vi "ScanSteuerung_LoopItAll.vi"(3 "needed constants":cluster{"AD-clock":dbl, "GalvoCycle":dbl}={"AD-clock"=4000000.0, "GalvoCycle"=1e-05}, 4 "ScanSteuerung":T1=[{"Time [s]"=0.0, "action"=enum."Abs", "channel"=enum."GalvoX", "value (/s)"=-8.3466666667e-05}, {"Time [s]"=0.0, "action"=enum."Abs", "channel"=enum."GalvoY", "value (/s)"=6.7466666667e-05}, {"Time [s]"=0.0, "action"=enum."Inc", "channel"=enum."GalvoX", "value (/s)"=0.0888}, {"Time [s]"=0.0, "action"=enum."Inc", "channel"=enum."GalvoY", "value (/s)"=0.0}, {"Time [s]"=0.00119, "action"=enum."LoopStart", "channel"=enum."Loop", "value (/s)"=4.0}, {"Time [s]"=0.00119, "action"=enum."Abs", "channel"=enum."Digital", "value (/s)"=7.0}, {"Time [s]"=0.002, "action"=enum."Inc", "channel"=enum."GalvoX", "value (/s)"=-3.3095271315e-17}, {"Time [s]"=0.002, "action"=enum."Inc", "channel"=enum."GalvoY", "value (/s)"=-0.0818}, {"Time [s]"=0.0022, "action"=enum."Inc", "channel"=enum."GalvoX", "value (/s)"=-0.0888}, {"Time [s]"=0.0022, "action"=enum."Inc", "channel"=enum."GalvoY", "value (/s)"=0.0}, {"Time [s]"=0.00319, "action"=enum."Abs", "channel"=enum."Digital", "value (/s)"=5.0}, {"Time [s]"=0.0033900000000000002, "action"=enum."Abs", "channel"=enum."Digital", "value (/s)"=7.0}, {"Time [s]"=0.0042, "action"=enum."Inc", "channel"=enum."GalvoX", "value (/s)"=3.3095271315e-17}, {"Time [s]"=0.0042, "action"=enum."Inc", "channel"=enum."GalvoY", "value (/s)"=-0.0818}, {"Time [s]"=0.0044, "action"=enum."Inc", "channel"=enum."GalvoX", "value (/s)"=0.0888}, {"Time [s]"=0.0044, "action"=enum."Inc", "channel"=enum."GalvoY", "value (/s)"=0.0}, {"Time [s]"=0.00539, "action"=enum."Abs", "channel"=enum."Digital", "value (/s)"=5.0}, {"Time [s]"=0.00559, "action"=enum."LoopEnd", "channel"=enum."Loop", "value (/s)"=0.0}, {"Time [s]"=0.01879, "action"=enum."Abs", "channel"=enum."Digital", "value (/s)"=7.0}, {"Time [s]"=0.0196, "action"=enum."Inc", "channel"=enum."GalvoX", "value (/s)"=-3.3095271315e-17}, {"Time [s]"=0.0196, "action"=enum."Inc", "channel"=enum."GalvoY", "value (/s)"=-0.0818}, {"Time [s]"=0.0198, "action"=enum."Inc", "channel"=enum."GalvoX", "value (/s)"=-0.0888}, {"Time [s]"=0.0198, "action"=enum."Inc", "channel"=enum."GalvoY", "value (/s)"=0.0}, {"Time [s]"=0.02079, "action"=enum."Abs", "channel"=enum."Digital", "value (/s)"=5.0}, {"Time [s]"=0.02099, "action"=enum."Abs", "channel"=enum."Digital", "value (/s)"=7.0}, {"Time [s]"=0.0218, "action"=enum."Inc", "channel"=enum."GalvoX", "value (/s)"=0.0}, {"Time [s]"=0.0218, "action"=enum."Inc", "channel"=enum."GalvoY", "value (/s)"=0.0}, {"Time [s]"=0.02299, "action"=enum."Abs", "channel"=enum."Digital", "value (/s)"=0.0}], 5 "Times":u32=10) -> (0 "ScanSteuerungOut":T1=[{"Time [s]"=0.0, "action"=enum."Abs", "channel"=enum."SMoveTime", "value (/s)"=0.0008}, {"Time [s]"=0.0, "action"=enum."Abs", "channel"=enum."GalvoX", "value (/s)"=-0.0005000005}, {"Time [s]"=0.0, "action"=enum."Abs", "channel"=enum."GalvoY", "value (/s)"=-0.0005000005}, {"Time [s]"=0.0, "action"=enum."Abs", "channel"=enum."Galvo3", "value (/s)"=0.0}, {"Time [s]"=0.0, "action"=enum."LoopStart", "channel"=enum."Loop", "value (/s)"=10.0}, {"Time [s]"=0.0, "action"=enum."Inc", "channel"=enum."GalvoX", "value (/s)"=1.000001e-06}, {"Time [s]"=0.0, "action"=enum."Inc", "channel"=enum."GalvoY", "value (/s)"=0.0}, {"Time [s]"=0.0, "action"=enum."Inc", "channel"=enum."Galvo3", "value (/s)"=0.512}, {"Time [s]"=999.9999999999999, "action"=enum."Abs", "channel"=enum."Digital", "value (/s)"=1.0}, {"Time [s]"=999.9999999999999, "action"=enum."Inc", "channel"=enum."GalvoX", "value (/s)"=0.0}, {"Time [s]"=999.9999999999999, "action"=enum."Inc", "channel"=enum."GalvoY", "value (/s)"=6.25000625e-06}, {"Time [s]"=999.9999999999999, "action"=enum."Inc", "channel"=enum."Galvo3", "value (/s)"=0.0}, {"Time [s]"=1008.0, "action"=enum."Abs", "channel"=enum."Digital", "value (/s)"=0.0}, {"Time [s]"=1008.0, "action"=enum."Inc", "channel"=enum."GalvoX", "value (/s)"=-1.000001e-06}, {"Time [s]"=1008.0, "action"=enum."Inc", "channel"=enum."GalvoY", "value (/s)"=-0.0}, {"Time [s]"=1008.0, "action"=enum."Inc", "channel"=enum."Galvo3", "value (/s)"=-0.512}, {"Time [s]"=2008.0, "action"=enum."Abs", "channel"=enum."Digital", "value (/s)"=1.0}, {"Time [s]"=2008.0, "action"=enum."Inc", "channel"=enum."GalvoX", "value (/s)"=0.0}, {"Time [s]"=2008.0, "action"=enum."Inc", "channel"=enum."GalvoY", "value (/s)"=6.25000625e-06}, {"Time [s]"=2008.0, "action"=enum."Inc", "channel"=enum."Galvo3", "value (/s)"=0.0}, {"Time [s]"=2016.0, "action"=enum."Abs", "channel"=enum."Digital", "value (/s)"=0.0}, {"Time [s]"=2016.0, "action"=enum."LoopEnd", "channel"=enum."Loop", "value (/s)"=0.0}, {"Time [s]"=20160.0, "action"=enum."Inc", "channel"=enum."GalvoX", "value (/s)"=0.0}, {"Time [s]"=20160.0, "action"=enum."Inc", "channel"=enum."GalvoY", "value (/s)"=0.0}, {"Time [s]"=20160.0, "action"=enum."Inc", "channel"=enum."Galvo3", "value (/s)"=0.0}], 1 "Looptime (1 image)":dbl)   [LabVIEW 2011]
uses:
  ScanControl.ctl
  ScanControl_Action.ctl
  ScanControl_Channel.ctl
panel:
  out "next GalvoSyncTime T1+T2":dbl
  out "time of last galvo (t1)":dbl
  out "index last galvocomand":i32
  out "Total Time":dbl
  # "sync to galvotime and ADTime"
  # "vor inner loopstat biite ein digital=0!r"
  # "seems to work!!"
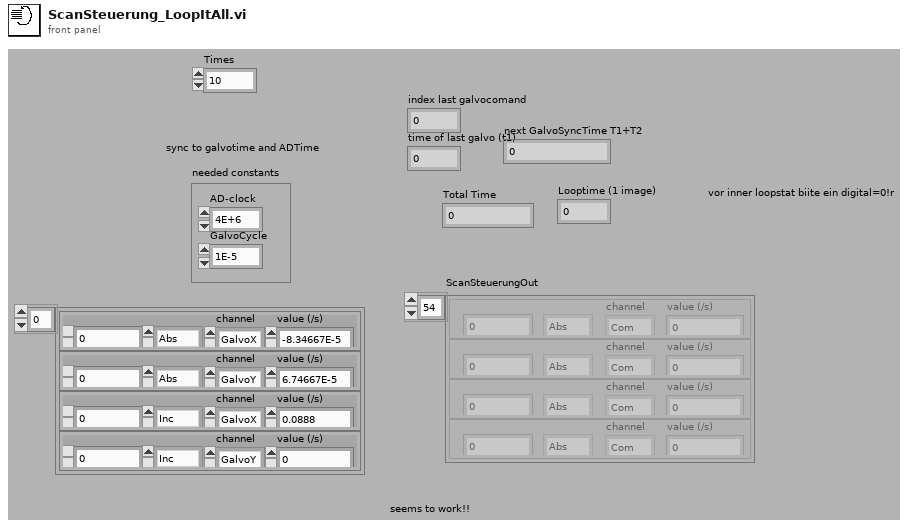
[diagram p1: front panel]
types:
  T1 = typedef "ScanControl.ctl" = cluster{"Time [s]":dbl, "action":T2, "channel":T3, "value (/s)":dbl}[]
  T2 = typedef "ScanControl_Action.ctl" = enum16{"Abs", "Rel", "Inc", "IncInc", "LoopStart", "LoopEnd", "WaitTriggerRising"}
  T3 = typedef "ScanControl_Channel.ctl" = enum16{"Com", "AnalogConfig", "AnalogValue", "GalvoX", "GalvoY", "Galvo3", "Galvo4", "Digital", "Free", "Loop", "SMoveTime", "Image1X", "Image1Y", "Image2X", "Image2Y"}
  T4 = enum16{"Com", "Digital", "Analog", "GalvoX", "GalvoY", "GalvoCCD", "Free1", "Free2", "Free3", "Loop", "SMoveTime", "Image1X", "Image1Y", "Image2X", "Image2Y"}
  T5 = enum16{"Com", "AnalogConfig", "AnalogValue", "GalvoX", "GalvoY", "Galvo3", "Galvo4", "Digital", "Free", "Loop", "SMoveTime", "Image1X", "Image1Y", "Image2X", "Image2Y"}
  T6 = enum16{"Abs", "Rel", "Inc", "IncInc", "LoopStart", "LoopEnd"}
  T7 = cluster{"Zeitpunkt [s]":dbl, "Wirkung":enum16{"Abs", "Rel", "Inc", "IncInc", "LoopStart", "LoopEnd"}, "Kanal":enum16{"Com", "AnalogConfig", "AnalogValue", "GalvoX", "GalvoY", "Galvo3", "Galvo4", "Digital", "Free", "Loop", "SMoveTime", "Image1X", "Image1Y", "Image2X", "Image2Y"}, "Wert (/s)":dbl}[]
  T8 = cluster{"Time [s]":dbl, "action":T2, "channel":T3, "value (/s)":dbl}
  T9 = cluster{"Time [s]":dbl, "Wirkung":enum16{"Abs", "Rel", "Inc", "IncInc", "LoopStart", "LoopEnd"}, "Kanal":enum16{"Com", "AnalogConfig", "AnalogValue", "GalvoX", "GalvoY", "Galvo3", "Galvo4", "Digital", "Free", "Loop", "SMoveTime", "Image1X", "Image1Y", "Image2X", "Image2Y"}, u32}
  T10 = cluster{dbl, "Wirkung":T2, "Kanal":enum16{"Com", "Digital", "Analog", "GalvoX", "GalvoY", "GalvoCCD", "Free1", "Free2", "Free3", "Loop", "SMoveTime", "Image1X", "Image1Y", "Image2X", "Image2Y"}, "Wert (/s)":dbl}
  T11 = cluster{"Time [s]":dbl, "action":T2, "Kanal":u16, "value (/s)":dbl}[]
  T12 = cluster{"Time [s]":dbl, "action":T2, "Kanal":u16, "value (/s)":dbl}
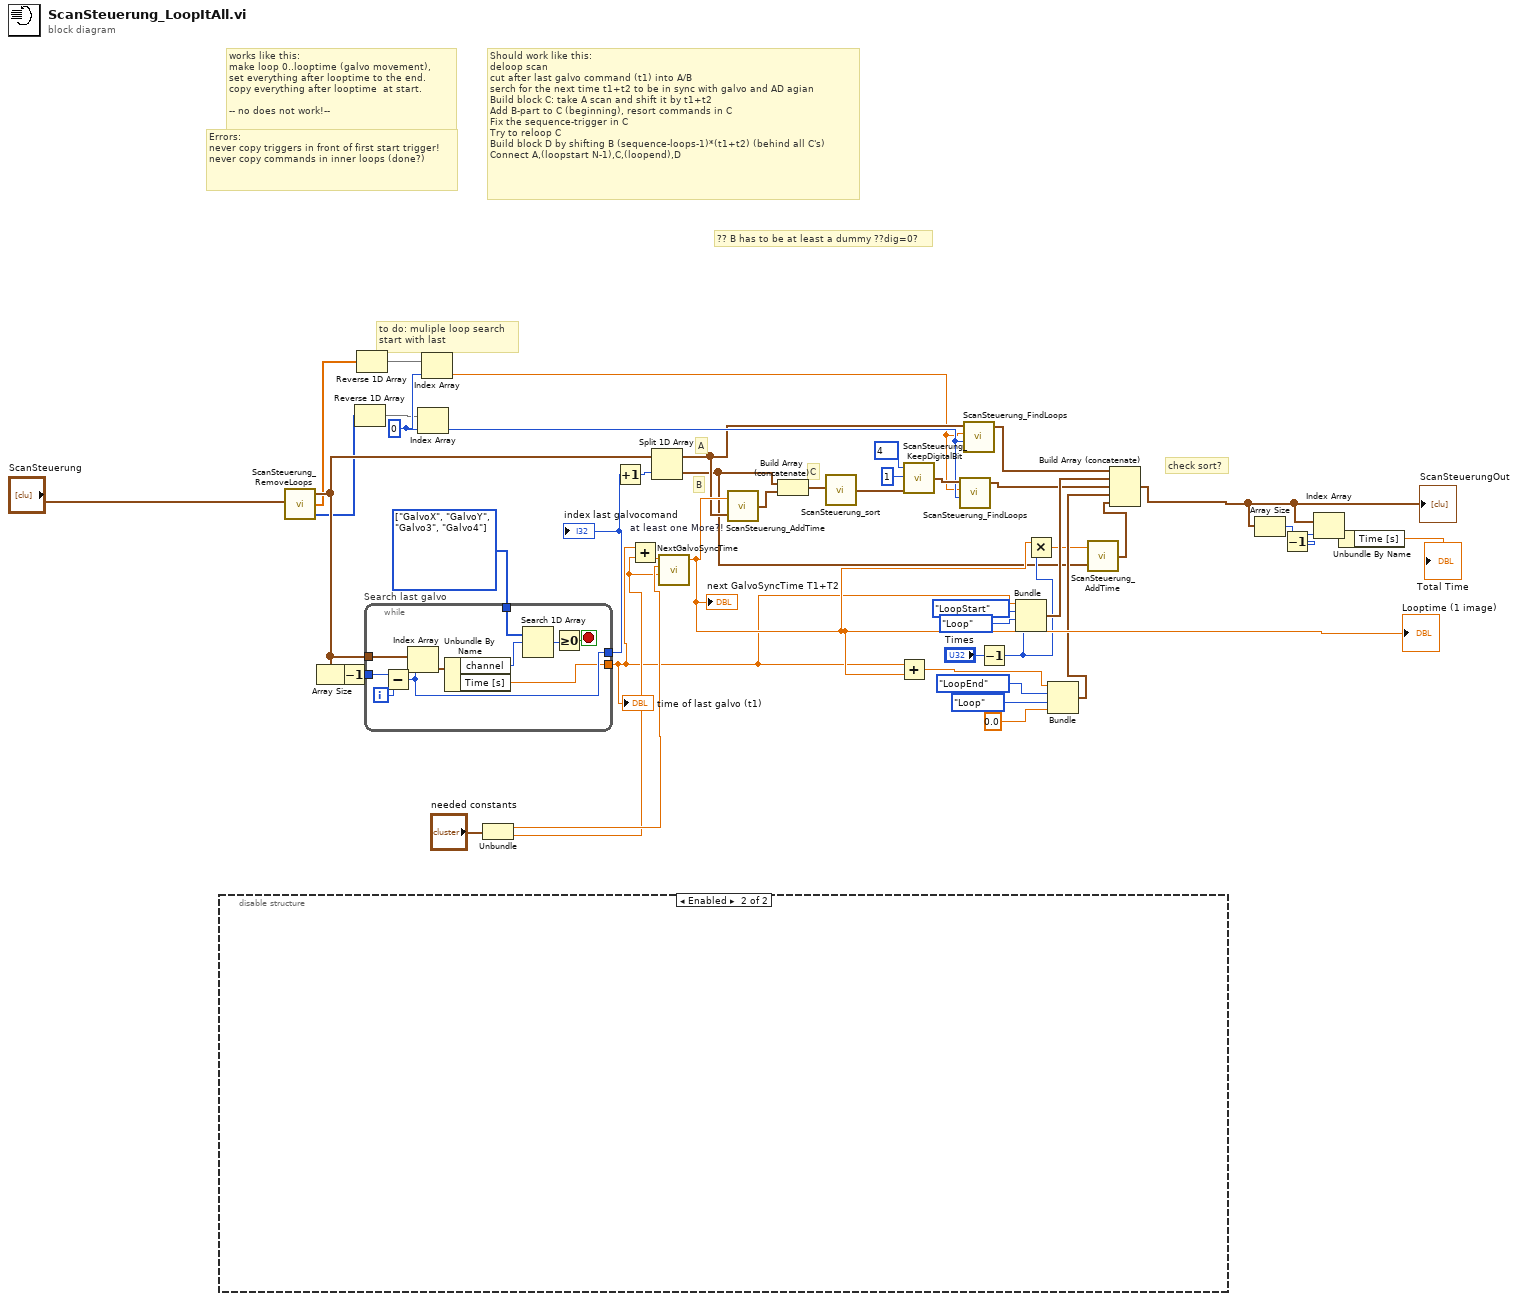
[diagram p0: block diagram]
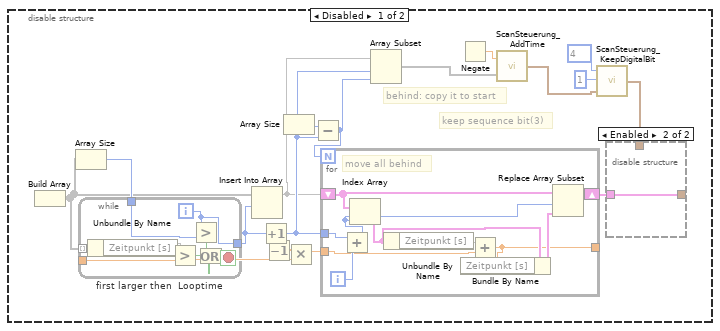
[diagram p2: hidden frame]
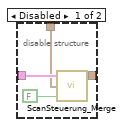
[diagram p3: hidden frame]
diagram:
  w3 = 0 ("index")
  w35 = T3[] [enum."GalvoX", enum."GalvoY", enum."Galvo3", enum."Galvo4"] items=["Com", "AnalogConfig", "AnalogValue", "GalvoX", "GalvoY", "Galvo3", "Galvo4", "Digital", "Free", "Loop", "SMoveTime", "Image1X", "Image1Y", "Image2X", "Image2Y"] ("1D array")
  # "check sort?"
  # "C"
  # "B"
  # "A"
  # "to do: muliple loop search\nstart with last"
  # "?? B has to be at least a dummy ??dig=0?"
  # "Errors:\nnever copy triggers in front of first start trigger!\nnever copy commands in inner loops (done?)"
  # "Should work like this:\ndeloop scan\ncut after last galvo command (t1) into A/B\nserch for the next time t1+t2 to be in sync with galvo and AD agian\nBuild block C: take A scan and shift it by t1+t2\nAdd B-part to C (beginning), resort commands in C\nFix the sequence-trigger in C\nTry to reloop C\nBuild block D by shifting B (sequence-loops-1)*(t1+t2) (behind all C's)\nConnect A,(loopstart N-1),C,(loopend),D"
  # "works like this: \nmake loop 0..looptime (galvo movement), \nset everything after looptime to the end.\ncopy everything after looptime  at start.\n\n-- no does not work!--"
  n1 = disable-structure shown="Enabled" {
    frame Disabled {
      # "keep sequence bit(3)"
      # "behind: copy it to start"
      n2 = Build Array() -> (w57:void[], w50:dbl, w51:dbl)
      n3 = Array Size(array=w57) -> (size(s)=w58:i32)
      n4 = Decrement() -> (x=w49:dbl, x-1=w56:dbl)
      n5 = Multiply(x=w56) -> (y=w64:dbl, x*y=w63:dbl)
      n6 = while "first larger then  Looptime" {
        tunnel: w57 -> [w93] mode=indexing
        tunnel: w64 -> [w91]
        tunnel: [w90] -> w54
        tunnel: w58 -> [w89]
        i -> [w90]
        stop <- w88 stop-if-true
        n7 = Unbundle By Name(w93) -> ("Zeitpunkt [s]"=w92)
        n8 = Greater?(x=w92, y=w91) -> (0:w87:bool)
        n9 = Greater?(x=w90, y=w89) -> (0:w86:bool)
        n10 = Or(x=w86, y=w87) -> (x .or. y?=w88:bool)
      }
      n11 = Insert Into Array(array=w57, index=w54) -> (w59, new element=w52:dbl)
      n12 = Increment(x=w54) -> (x+1=w61:i32)
      n13 = Array Size(array=w59) -> (size(s)=w53:i32)
      n14 = Subtract(x=w53, y=w61) -> (x-y=w60:i32)
      n15 = for {
        N: w60 -> [_]
        shift-right: [w82] -> w66
        shift-left: w59 -> [w83]
        tunnel: w63 -> [w80]
        tunnel: w61 -> [w85]
        tunnel: [w76] -> w55
        i -> [w84]
        # "move all behind"
        n16 = Add(x=w85, y=w84) -> (x+y=w77:i32)
        n17 = Index Array(array=w83, index=w77) -> (element=w79:cluster{})
        n18 = Unbundle By Name(w79) -> ("Zeitpunkt [s]"=w81)
        n19 = Add(x=w81, y=w80) -> (x+y=w76:dbl)
        n20 = Bundle By Name(cluster=w79, "Zeitpunkt [s]"=w76) -> (w78:cluster{})
        n21 = Replace Array Subset(array=w83, new element=w78, index=w77) -> (w82:cluster{}[])
      }
      n22 = Array Subset(array=w59, index=w61, length=w60) -> (w62:void[])
      n23 = Negate() -> (x=w48:dbl, -x=w65:dbl)
      n24 = call "ScanSteuerung_AddTime.vi"("ScanSteuerung"=w62, "Add Time"=w65) -> ("ScanSteuerungOut"=w67:T1)
      n25 = call "ScanSteuerung_KeepDigitalBit.vi"("ScanSteuerung"=w67, "Value (0/1)"=u8 1, "Bitmask"=u32 4) -> ("ScanSteuerungOut"=w68:T1)
      n26 = disable-structure shown="Enabled" {
        disable-tunnel: [w74 w75] -> _
        disable-tunnel: w66 -> [w73 w75]
        disable-tunnel: w68 -> [w71 _]
        frame Disabled {
          n27 = call "ScanSteuerung_Merge.vi"("if equal: insert later"=FALSE ("equal:later"), "Insert"=w71, "ScanControl"=w73) -> ("ScanSteuerungOut"=w74:T7)  [unwired: 2 out]
        }
        frame Enabled {
        }
      }
    }
    frame Enabled {
    }
  }
  n28 = call "ScanSteuerung_RemoveLoops.vi"("ScanSteuerung"="ScanSteuerung") -> ("ScanSteuerungOut"=w32:T1, "LoopLengths"=w5:dbl[], "Loopelements"=w25:i32[])
  n29 = Array Size(array=w32) -> (size(s)=w37:i32)
  n30 = Decrement(x=w37) -> (x-1=w36:i32)
  n31 = Reverse 1D Array(array=w25) -> (reversed array=w1:i32[])
  n32 = Reverse 1D Array(array=w5) -> (reversed array=w2:dbl[])
  n33 = while "Search last galvo" {
    tunnel: w32 -> [w101]
    tunnel: w36 -> [w103]
    tunnel: w35 -> [w98]
    tunnel: [w95] -> w34
    tunnel: [w94] -> w14
    i -> [w102]
    stop <- w96 stop-if-true
    n34 = Subtract(x=w103, y=w102) -> (x-y=w95:i32)
    n35 = Index Array(array=w101, index=w95) -> (element=w100:T8)
    n36 = Unbundle By Name(w100) -> ("channel"=w99:T3, "Time [s]"=w94:dbl)
    n37 = Search 1D Array(1D array=w98, element=w99) -> (index of element=w97:i32)  [unwired: 1 out]
    n38 = Greater Or Equal To 0?(x=w97) -> (x >= 0?=w96:bool)
  }
  "index last galvocomand" <- w34
  "time of last galvo (t1)" <- w14
  n39 = Index Array(array=w1, index=w3) -> (element=w8:i32)
  n40 = Index Array(array=w2, index=w3) -> (element=w4:dbl)
  n41 = Unbundle("needed constants") -> ("AD-clock"=w39:dbl, "GalvoCycle"=w38:dbl)
  n42 = Increment(x=w34) -> (x+1=w33:i32)
  n43 = Add "at least one More?!"(x=w14, y=w38) -> (x+y=w15:dbl)
  n44 = Split 1D Array(array=w32, index=w33) -> (first subarray=w7:T1, second subarray=w6:T1)
  n45 = call "NextGalvoSyncTime.vi"("Galvocycle [s]"=w38, "AD-Frquency [Hz]"=w39, "Timepoint"=w15) -> ("next GalvoSyncTime"=w46:dbl)  [unwired: 1 in, 2 out]
  "Looptime (1 image)" <- w46
  "next GalvoSyncTime T1+T2" <- w46
  n46 = call "ScanSteuerung_AddTime.vi"("ScanSteuerung"=w7, "Add Time"=w46) -> ("ScanSteuerungOut"=w31:T1)
  n47 = Build Array (concatenate)(w6, w31) -> (w30:T1)
  n48 = call "ScanSteuerung_sort.vi"("ScanSteuerung"=w30) -> ("ScanSteuerung"=w27:T1)
  n49 = Add(x=w14, y=w46) -> (x+y=w13:dbl)
  n50 = call "ScanSteuerung_KeepDigitalBit.vi"("ScanSteuerung"=w27, "Value (0/1)"=u8 1, "Bitmask"=u32 4) -> ("ScanSteuerungOut"=w26:T1)
  n51 = call "ScanSteuerung_FindLoops.vi"("LoopElements"=w8, "Looptime"=w4, "ScanSteuerung"=w26) -> ("ScanSteuerungOut"=w20:T1)  [unwired: 1 in, 2 out]
  n52 = call "ScanSteuerung_FindLoops.vi"("LoopElements"=w8, "Looptime"=w4, "ScanSteuerung"=w7) -> ("ScanSteuerungOut"=w9:T1)  [unwired: 1 in, 2 out]
  n53 = Decrement(x="Times") -> (x-1=w12:u32)
  n54 = Bundle("Time [s]"=w14, "Wirkung"=T6."LoopStart", "Kanal"=T5."Loop", w12) -> (w21:T9)  [unwired: 1 out]
  n55 = Multiply(x=w46, y=w12) -> (x*y=w11:dbl)
  n56 = Bundle(w13, "Wirkung"=ScanControl_Action."LoopEnd", "Kanal"=T4."Loop", "Wert (/s)"=0.0) -> (w16:T10)  [unwired: 1 out]
  n57 = call "ScanSteuerung_AddTime.vi"("ScanSteuerung"=w6, "Add Time"=w11) -> ("ScanSteuerungOut"=w10:T1)
  n58 = Build Array (concatenate)(w9, w21, w20, w16, w10) -> (w45:T11)
  "ScanSteuerungOut" <- w45
  n59 = Array Size(array=w45) -> (size(s)=w44:i32)
  n60 = Decrement(x=w44) -> (x-1=w43:i32)
  n61 = Index Array(array=w45, index=w43) -> (element=w42:T12)
  n62 = Unbundle By Name(w42) -> ("Time [s]"=→"Total Time":dbl)
